vi "UI_Start Test Wizard.vi"(6 "error in (no error)":errorcluster, 9 "Full Config":T2={"Bench Params"={"Relative Root Name"="", "Values"={"Step Levels"=0.0, "Resistor Tolerence"=0.0, "Sample Rate"=0.0, "Resistor"=0.0, "Wait Time"=0.0}, "Report Template path"=path "$ReportFiles/ReportTemplate_03.xlsx", "Test Type"="", "Config File Name"="", "Config 2 Use"="", "Skip Pre Lube"=FALSE}, "Test Params"=[], "Pump Params"={"Empty Inches"=0.0, "Full Inches"=0.0, "RNG_SLOW"=0.0, "RNG_CREEP"=0.0, "RNG_STOP "=0.0, "VISA resource name"="", "SPD_SLOW"=0, "SPD_CREEP"=0, "SPD_FAST"=0, "Zero template"=path "", "zero  Settle sec"=0, "Laser Slope"=0.0, "Laser Offset"=0.0, "Sim Fill Rate"=0.0, "Cal Date"="", "Cal Technician"=""}, "DataQ Params"={"Visa Name"="", "Num Chan"=0, "Cal Coef"=[], "Scale "=0, "Cal Date"="", "Cal Technicain"=""}, "Pump Control Ref"={"Fill "=refnum, "Drain"=refnum, "Level PV"=refnum, "Pump Speed"=refnum, "Run Test"=refnum, "Sim"=refnum, "Jog"=refnum, "Level SP"=refnum}, "Bench Status"={"Pump Status"=refnum, "Instrumnet\n Status"=refnum}} {"Pump Params"."Sim Fill Rate" format="%.3f"; "Pump Params"."Laser Offset" format="%.3f"; "Pump Params"."Laser Slope" format="%.3f"; "Pump Params"."RNG_STOP" format="%#_13g"; "Pump Params"."RNG_CREEP" format="%#_13g"; "Pump Params"."RNG_SLOW" format="%#_13g"}) -> (0 "error out":errorcluster, 1 "Time Base mS":i32, 2 "Title":string, 3 "Sample Rate":dbl, 4 "Test Info":T1={"Job Number"="", "Unit Number"="", "Serial Number"="", "Technician Name"="", "Calibration Date"="Cal Date", "Calibrator"="Cal by", "Calibration Slope"="M", "Calibration Offset"="B", "Config File Name"="Cal Date"})   [LabVIEW 2024]
uses:
  Control Definitions/DEF_FullConfig.ctl
  Control Definitions/DEF_BenchParams.ctl
  Control Definitions/DEF_PumpParams.ctl
  Control Definitions/DEF_DataqParams.ctl
  Control Definitions/DEF_PumpCtlRefs.ctl
  Control Definitions/Def_PumpSpeed.ctl
  Control Definitions/DEF_BenchStatus.ctl
  Control Definitions/DEF_TestInfo.ctl
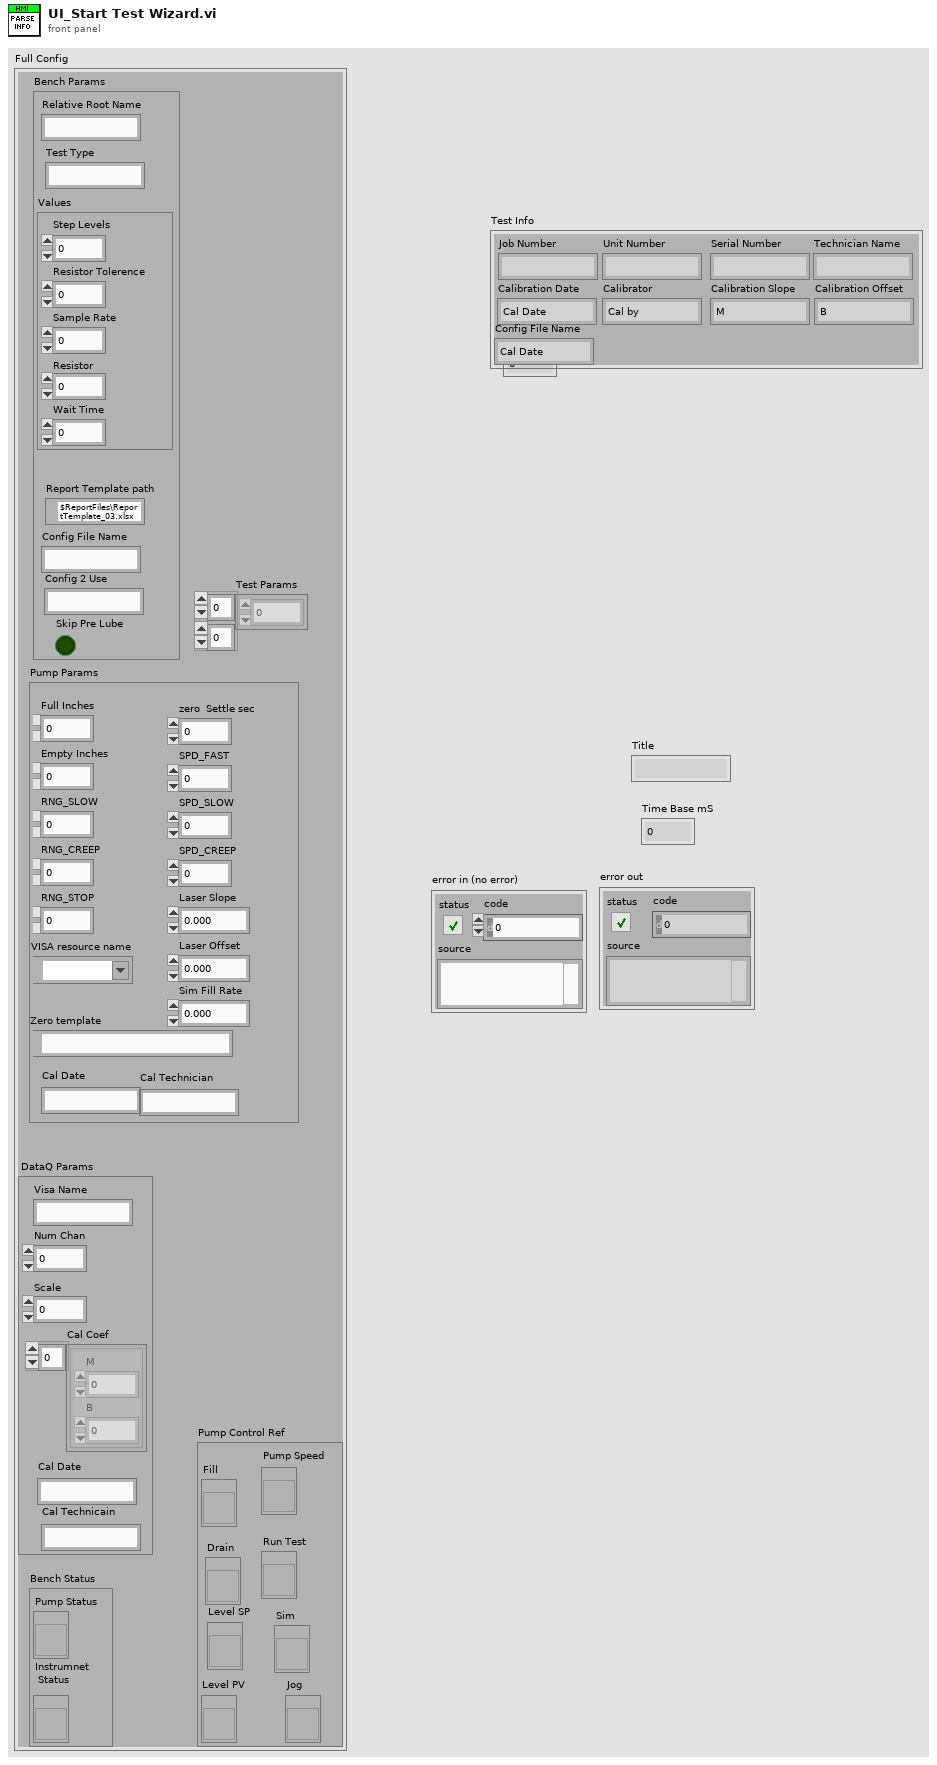
[diagram p1: front panel]
types:
  T1 = typedef "DEF_TestInfo.ctl" = cluster{"Job Number":string, "Unit Number":string, "Serial Number":string, "Technician Name":string, "Calibration Date":string, "Calibrator":string, "Calibration Slope":string, "Calibration Offset":string, "Config File Name":string}
  T2 = typedef "DEF_FullConfig.ctl" = cluster{"Bench Params":T3, "Test Params":dbl[][], "Pump Params":T4, "DataQ Params":T5, "Pump Control Ref":T6, "Bench Status":T7}
  T3 = typedef "DEF_BenchParams.ctl" = cluster{"Relative Root Name":string, "Values":cluster{"Step Levels":dbl, "Resistor Tolerence":dbl, "Sample Rate":dbl, "Resistor":dbl, "Wait Time":dbl}, "Report Template path":path, "Test Type":string, "Config File Name":string, "Config 2 Use":string, "Skip Pre Lube":bool}
  T4 = typedef "DEF_PumpParams.ctl" = cluster{"Empty Inches":dbl, "Full Inches":dbl, "RNG_SLOW":dbl, "RNG_CREEP":dbl, "RNG_STOP ":dbl, "VISA resource name":refnum<visa-resource-name>, "SPD_SLOW":i32, "SPD_CREEP":i32, "SPD_FAST":i32, "Zero template":path, "zero  Settle sec":i32, "Laser Slope":sgl, "Laser Offset":sgl, "Sim Fill Rate":sgl, "Cal Date":string, "Cal Technician":string}
  T5 = typedef "DEF_DataqParams.ctl" = cluster{"Visa Name":string, "Num Chan":i32, "Cal Coef":cluster{"M":dbl, "B":dbl}[], "Scale ":i32, "Cal Date":string, "Cal Technicain":string}
  T6 = typedef "DEF_PumpCtlRefs.ctl" = cluster{"Fill ":refnum<vi>, "Drain":refnum<vi>, "Level PV":refnum<vi>, "Pump Speed":refnum<vi>, "Run Test":refnum<vi>, "Sim":refnum<vi>, "Jog":refnum<vi>, "Level SP":refnum<vi>}
  T7 = typedef "DEF_BenchStatus.ctl" = cluster{"Pump Status":refnum<vi>, "Instrumnet\n Status":refnum<vi>}
  T8 = typedef "Def_PumpSpeed.ctl" = enum16{"FAST", "SLOW", "CREEP", "STOP"}
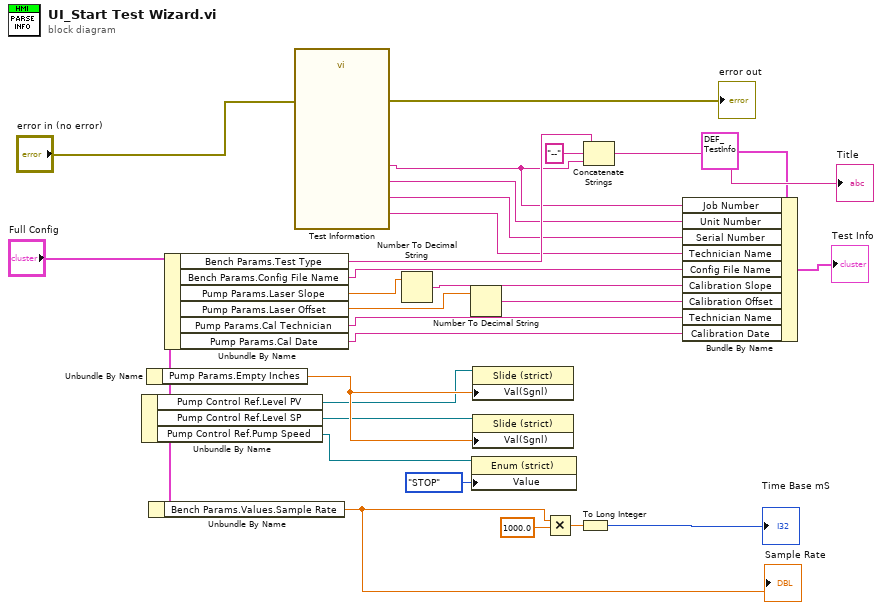
[diagram p0: block diagram]
diagram:
  n1 = Unbundle By Name("Full Config") -> ("Pump Control Ref.Level PV"=w13:refnum<vi>, "Pump Control Ref.Level SP"=w12:refnum<vi>, "Pump Control Ref.Pump Speed"=w2:refnum<vi>)
  n2 = Unbundle By Name("Full Config") -> ("Pump Params.Empty Inches"=w15:dbl)
  n3 = Unbundle By Name("Full Config") -> ("Bench Params.Values.Sample Rate"=w14:dbl)
  "Sample Rate" <- w14
  n4 = Unbundle By Name("Full Config") -> ("Bench Params.Test Type"=w21:string, "Bench Params.Config File Name"=w9:string, "Pump Params.Laser Slope"=w6:sgl, "Pump Params.Laser Offset"=w4:sgl, "Pump Params.Cal Technician"=w8:string, "Pump Params.Cal Date"=w7:string)
  n5 = call "Test Information"("error in (no error)"="error in (no error)") -> ("Technician Name"=w17:string, "Serial Number"=w18:string, "Unit Number"=w19:string, "Job Number"=w20:string, "error out"=→"error out":errorcluster)  [unwired: 13 in, 1 out]
  n6 = Number To Decimal String(number=w6) -> (decimal integer string=w5:string)  [unwired: 1 in]
  n7 = Number To Decimal String(number=w4) -> (decimal integer string=w3:string)  [unwired: 1 in]
  n8 = property class="Enum (strict)"(reference=w2, "Value"=Def_PumpSpeed."STOP") -> ()  [unwired: 1 in, 2 out]
  n9 = property on="Property Node" class="Slide (strict)"(reference=w13, "Val(Sgnl)"=w15) -> ()  [unwired: 1 in, 2 out]
  n10 = property on="Property Node" class="Slide (strict)"(reference=w12, "Val(Sgnl)"=w15) -> ()  [unwired: 1 in, 2 out]
  n11 = Multiply(x=w14, y=1000.0) -> (x*y=w26:dbl)
  n12 = To Long Integer(number=w26) -> (32bit integer=→"Time Base mS":i32)
  n13 = Concatenate Strings(w21, "--" ("string"), w20) -> (→"Title":string)
  n14 = Bundle By Name(cluster=T1 {"Job Number"="", "Unit Number"="", "Serial Number"="", "Technician Name"="", "Calibration Date"="Cal Date", "Calibrator"="Cal by", "Calibration Slope"="M", "Calibration Offset"="B", "Config File Name"="Cal Date"} ("Test Info"), "Job Number"=w20, "Unit Number"=w19, "Serial Number"=w18, "Technician Name"=w17, "Config File Name"=w9, "Calibration Slope"=w5, "Calibration Offset"=w3, "Technician Name"=w8, "Calibration Date"=w7) -> (→"Test Info":T1)
